vi "Test App Get All Processes Twice.vi"(8 "error in (no error)":errorcluster, 11 "Rig Test in":refnum<class "Application Test.lvclass">) -> (0 "error out":errorcluster, 3 "Rig Test out":refnum<class "Application Test.lvclass">)   [LabVIEW 2020, in "Application Test.lvclass"]
uses:
  Application Test.lvclass
  Framework/Process/Process.lvclass
  Framework/Application/Application.lvclass
  C:/Users/anton/Documents/GitHub/Triarc-Framework/source/Framework/Process/Process.lvclass
  C:/Users/anton/Documents/GitHub/Triarc-Framework/source/Framework/Base/Base.lvclass
  C:/Users/anton/Documents/GitHub/Triarc-Framework/source/Framework/Error Handler Interface/Error Handler Interface.lvclass
  C:/Users/anton/Documents/GitHub/Triarc-Framework/source/Framework/Logging/Logging.lvclass
  C:/Users/anton/Documents/GitHub/Triarc-Framework/source/Framework/Application/Application.lvclass
  C:/Users/anton/Documents/GitHub/Triarc-Framework/source/Framework/Asynchronous Action/Async Action.lvclass
  <vilib>/Asteme/LUnit/Test Case.lvclass
  C:/Users/anton/Documents/GitHub/Triarc-Framework/source/Framework Test/Process Test/Process Test.lvclass
  C:/Users/anton/Documents/GitHub/Triarc-Framework/source/Framework Test/Base Class Test/Base Test.lvclass
  C:/Program Files (x86)/National Instruments/LabVIEW 2020/vi.lib/Asteme/LUnit/Test Case.lvclass
  C:/Users/anton/Documents/GitHub/Triarc-Framework/source/Framework Test/Application Test/Application Test.lvclass
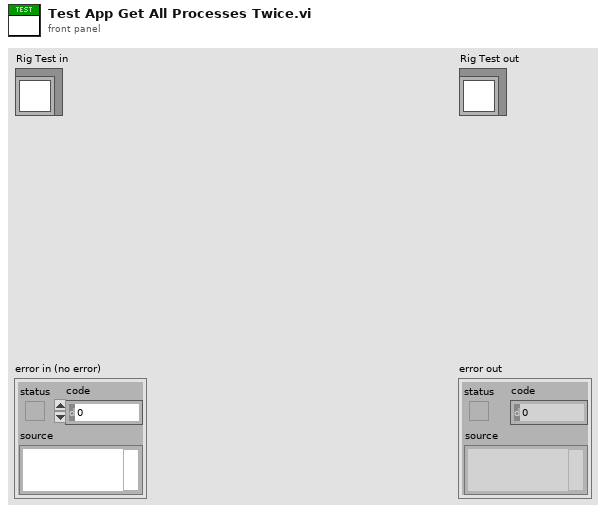
[diagram p1: front panel]
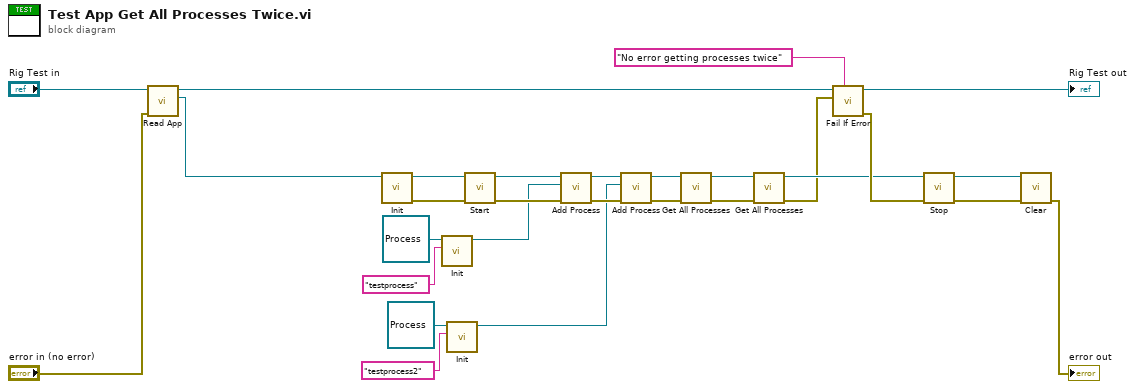
[diagram p0: block diagram]
diagram:
  n1 = call "Read App.vi"("error in (no error)"="error in (no error)", "Application Test In"="Rig Test in") -> ("App out"=w27:refnum<class "Application.lvclass">, "Application Test Out"=w15:refnum<class "Application Test.lvclass">)  [unwired: 7 in, 1 out]
  n2 = call-dynamic "Init.vi"("Process In"=w27) -> ("error out"=w16:errorcluster, "Process Out"=w17:refnum<class "Application.lvclass">)  [unwired: 9 in]
  n3 = call-dynamic "Init.vi"("Name"="testprocess", "Process In"=refnum<class "Process.lvclass"> refnum ("Process.lvclass")) -> ("Process Out"=w14:refnum<class "Process.lvclass">)  [unwired: 8 in, 1 out]
  n4 = call-dynamic "Init.vi"("Name"="testprocess2", "Process In"=refnum<class "Process.lvclass"> refnum ("Process.lvclass")) -> ("Process Out"=w4:refnum<class "Process.lvclass">)  [unwired: 8 in, 1 out]
  n5 = call "Start.vi"("error in (no error)"=w16, "Process In"=w17) -> ("error out"=w18:errorcluster, "Process Out"=w19:refnum<class "Application.lvclass">)  [unwired: 8 in]
  n6 = call "Add Process.vi"("error in (no error)"=w18, "Process"=w14, "Rig In"=w19) -> ("error out"=w23:errorcluster, "Rig Out"=w9:refnum<class "Application.lvclass">)  [unwired: 7 in]
  n7 = call "Add Process.vi"("error in (no error)"=w23, "Process"=w4, "Rig In"=w9) -> ("error out"=w10:errorcluster, "Rig Out"=w8:refnum<class "Application.lvclass">)  [unwired: 7 in]
  n8 = call "Get All Processes.vi"("error in (no error)"=w10, "Application In"=w8) -> ("error out"=w6:errorcluster, "Application Out"=w3:refnum<class "Application.lvclass">)  [unwired: 7 in, 1 out]
  n9 = call "Get All Processes.vi"("error in (no error)"=w6, "Application In"=w3) -> ("error out"=w1:errorcluster, "Application Out"=w2:refnum<class "Application.lvclass">)  [unwired: 7 in, 1 out]
  n10 = call <vilib>:"Fail If Error.vi"("Description"="No error getting processes twice", "Assert error"=w1, "Test Case In"=w15) -> ("error out"=w21:errorcluster, "Test Case Out"=→"Rig Test out":refnum<class "Application Test.lvclass">)  [unwired: 7 in]
  n11 = call "Stop.vi"("error in (no error)"=w21, "Process In"=w2) -> ("error out"=w13:errorcluster, "Process Out"=w12:refnum<class "Application.lvclass">)  [unwired: 7 in, 1 out]
  n12 = call-dynamic "Clear.vi"("error in (no error)"=w13, "Application In"=w12) -> ("error out"=→"error out":errorcluster)  [unwired: 9 in]
